vi "InstrPtr Demo.vi"   [LabVIEW 2009]
uses:
  Instrument/Instrument.lvclass
  InstrPtr.lvclass
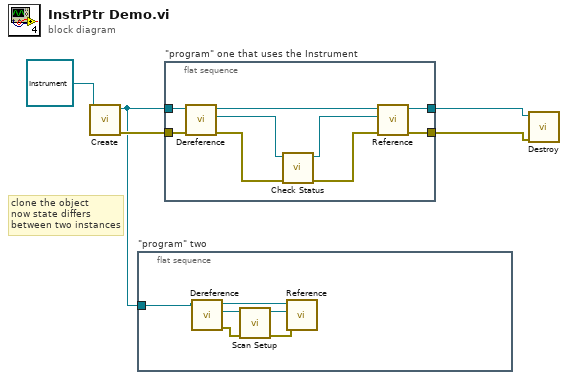
[diagram p0: block diagram]
diagram:
  # "clone the object\nnow state differs \nbetween two instances"
  n1 = call "Create.vi"("Instrument in"=refnum<class "Instrument.lvclass"> refnum) -> ("error out"=w5:errorcluster, "InstrPtr out"=w3:refnum<class "InstrPtr.lvclass">)  [unwired: 2 in, 7 out]
  n2 = flat-sequence "\"program\" two" {
    tunnel: w3 -> [w9]
    frame #0 {
      n3 = call-dynamic "Dereference.vi"("InstrPtr in"=w9) -> ("error out"=w11:errorcluster, "Instrument"=w10:refnum<class "Instrument.lvclass">, "InstrPtr out"=w8:refnum<class "InstrPtr.lvclass">)  [unwired: 1 in, 7 out]
      n4 = call-dynamic "Scan Setup.vi"("error in (no error)"=w11, "Instrument in"=w10) -> ("error out"=w6:errorcluster, "Instrument out"=w7:refnum<class "Instrument.lvclass">)  [unwired: 8 out]
      n5 = call-dynamic "Reference.vi"("error in (no error)"=w6, "Instrument"=w7, "InstrPtr in"=w8) -> ()  [unwired: 9 out]
    }
  }
  n6 = flat-sequence "\"program\" one that uses the Instrument" {
    tunnel: w3 -> [w19]
    tunnel: w5 -> [w18]
    tunnel: [w13] -> w2
    tunnel: [w12] -> w1
    frame #0 {
      n7 = call-dynamic "Dereference.vi"("error in (no error)"=w18, "InstrPtr in"=w19) -> ("error out"=w15:errorcluster, "Instrument"=w17:refnum<class "Instrument.lvclass">, "InstrPtr out"=w20:refnum<class "InstrPtr.lvclass">)  [unwired: 7 out]
      n8 = call-dynamic "Check Status.vi"("error in (no error)"=w15, "Instrument in"=w17) -> ("error out"=w14:errorcluster, "Instrument out"=w16:refnum<class "Instrument.lvclass">)  [unwired: 8 out]
      n9 = call-dynamic "Reference.vi"("error in (no error)"=w14, "Instrument"=w16, "InstrPtr in"=w20) -> ("error out"=w12:errorcluster, "InstrPtr out"=w13:refnum<class "InstrPtr.lvclass">)  [unwired: 7 out]
    }
  }
  n10 = call "Destroy.vi"("error in (no error)"=w1, "InstrPtr in"=w2) -> ()  [unwired: 1 in, 9 out]
